vi "Init Array of CCD monitor Config Objs.vi"(8 "error in (no error)":errorcluster, 11 "Hardware.lvlib:CCD monitor.lvlib:CCD monitor configuration.lvclass":refnum<class "CCD monitor configuration.lvclass">) -> (0 "error out":errorcluster, 2 "Array of CCD monitor":refnum<class "CCD Configuration.lvclass">[](array[class]), 3 "reference out":refnum<class "CCD monitor configuration.lvclass">)   [LabVIEW 2016, in "CCD monitor.lvlib" / "CCD monitor configuration.lvclass"]
uses:
  <userlib>/Common Components/Hardware/Abstract System/Monitor/CCD monitor configuration.lvclass
  <userlib>/Common Components/Hardware/Abstract System/Monitor/CCD monitor.lvclass
  <userlib>/Common Components/Hardware/CCD/CCD Configuration.lvclass
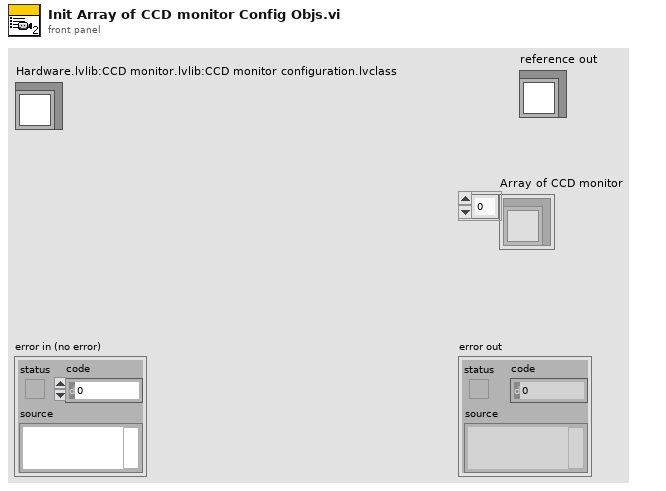
[diagram p1: front panel]
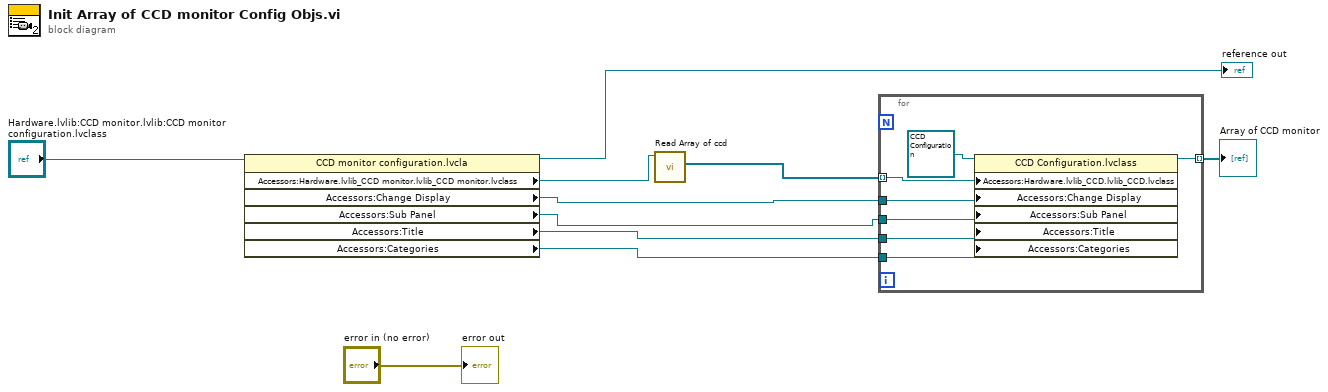
[diagram p0: block diagram]
diagram:
  n1 = property class="CCD monitor configuration.lvcla"(reference="Hardware.lvlib:CCD monitor.lvlib:CCD monitor configuration.lvclass") -> (reference out=→"reference out":refnum<class "CCD monitor configuration.lvclass">, "Accessors:Hardware.lvlib_CCD monitor.lvlib_CCD monitor.lvclass"=w4:refnum<class "CCD monitor.lvclass">, "Accessors:Change Display"=w9:refnum<user-event>, "Accessors:Sub Panel"=w8:refnum<vi>, "Accessors:Title"=w7:refnum<vi>, "Accessors:Categories"=w6:refnum<vi>)  [unwired: 1 in, 1 out]
  n2 = call <userlib>:"Read Array of ccd.vi"("CCD monitor in"=w4) -> ("Array of ccd"=w3:refnum<class "CCD.lvclass">[])  [unwired: 9 in, 1 out]
  n3 = for {
    tunnel: w9 -> [w17]
    tunnel: w8 -> [w16]
    tunnel: w7 -> [w15]
    tunnel: w6 -> [w14]
    tunnel: [w13] -> w2 mode=indexing
    tunnel: w3 -> [w11] mode=indexing
    n4 = property class="CCD Configuration.lvclass"(reference=refnum<class "CCD Configuration.lvclass"> refnum ("Hardware.lvlib:CCD.lvlib:CCD Configuration.lvclass"), "Accessors:Hardware.lvlib_CCD.lvlib_CCD.lvclass"=w11, "Accessors:Change Display"=w17, "Accessors:Sub Panel"=w16, "Accessors:Title"=w15, "Accessors:Categories"=w14) -> (reference out=w13:refnum<class "CCD Configuration.lvclass">)  [unwired: 1 in, 1 out]
  }
  "Array of CCD monitor" <- w2
  "error out" <- "error in (no error)"
